vi "Lvi Set Reference Trigger.vi"(5 "ThresholdChannel":u32, 6 "AnalogThreshold":dbl, 7 "NumSamples":u32, 8 "error in (no error)":errorcluster, 9 "Polarity":i32, 10 "TrigType":i32, 11 "TaskRef":i32) -> (0 "error out":errorcluster, 2 "function return":i32, 3 "TaskRef out":i32)   [LabVIEW 2022 SP3, in "DtLvLink.lvlib"]
doc: "Calls directly into the entry points of the DLL of the Data Acq SDK to specify the attributes of the reference trigger for an analog input task. This VI is used by the higher-level VI, DtOLTrigger."
uses:
  DtLvLink.lvlib
  <userlib>/LV-Link3/DtLvLink_64.dll
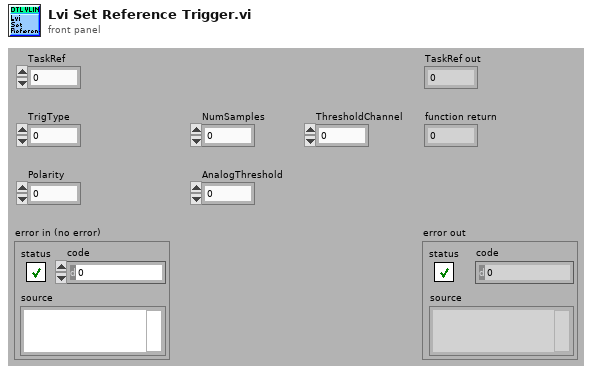
[diagram p1: front panel]
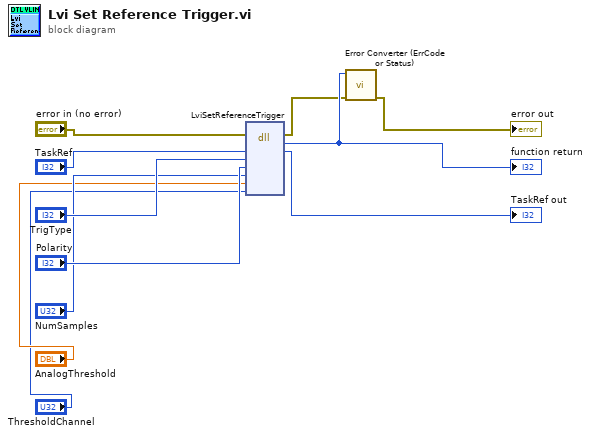
[diagram p0: block diagram]
diagram:
  n1 = dll-call lib="C:/Program Files/National Instruments/LabVIEW 2022/user.lib/LV-Link3/DtLvLink_64.*" fn="LviSetReferenceTrigger"(error in="error in (no error)", "TaskRef"="TaskRef", "TrigType"="TrigType", "Polarity"="Polarity", "NumSamples"="NumSamples", "AnalogThreshold"="AnalogThreshold", "ThresholdChannel"="ThresholdChannel") -> (error out=w2:errorcluster, "return type"=w11:i32, "TaskRef"=→"TaskRef out":i32)  [unwired: 7 in, 1 out]
  "function return" <- w11
  n2 = call "Error Converter (ErrCode or Status).vi"("error in (no error)"=w2, "error code"=w11) -> ("error out"=→"error out":errorcluster)  [unwired: 9 in]
